vi "Element by Hierarchy.vi"(8 "error in (no error)":errorcluster, 10 "Hierarchy":string[](array[string]), 11 "Config Manager in":refnum<class "Config Manager.lvclass">) -> (0 "error out":errorcluster, 2 "Config Element":refnum<class "Config Element.lvclass">, 3 "Config Manager out":refnum<class "Config Manager.lvclass">)   [LabVIEW 2020, in "CDM-Config.lvlib" / "Config Manager.lvclass"]
doc: "Returns the specified element or an error if the specified hierarchy name does not exist. If the specified hierarchy is empty, the root element is returned."
uses:
  Config Manager.lvclass
  CDM-Config.lvlib
  Config Element/Config Element.lvclass
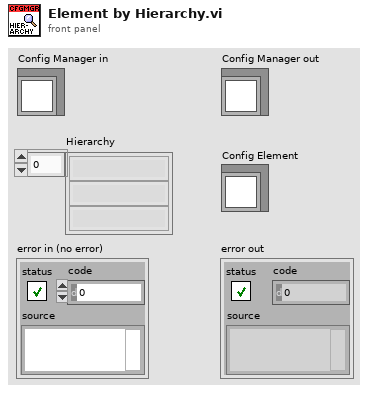
[diagram p1: front panel]
types:
  T1 = typedef "CDM-Config.lvlib/Config Manager.lvclass/Ref Data.ctl" = cluster{"Elements":refnum<class "Config Element.lvclass">[], "Hierarchy Map":map{string[], i32}, "Element Map":map{refnum<class "Config Element.lvclass">, i32}}
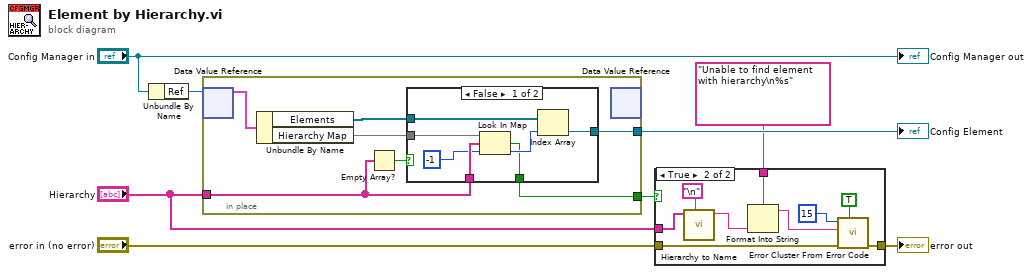
[diagram p0: block diagram]
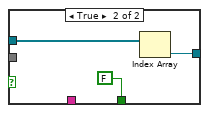
[diagram p2: hidden frame]
diagram:
  n1 = Unbundle By Name("Config Manager in") -> ("Ref"=w7:refnum<data-value>)
  n2 = in-place {
    in-place-border: "Hierarchy" -> [w9]
    in-place-border: [w12] -> w6
    in-place-border: [w11] -> w4
    n3 = in-place-dvr #1(w7) -> (w15:T1)  [unwired: 1 out]
    n4 = Unbundle By Name(w15) -> ("Elements"=w13:refnum<class "Config Element.lvclass">[], "Hierarchy Map"=w14:map{string[], i32})
    n5 = Empty Array?(array=w9) -> (empty?=w10:bool)
    n6 = case shown="False" w10 {
      tunnel: w14 -> [w22 _]
      tunnel: w13 -> [w21 w24]
      tunnel: [w19 w23] -> w12
      tunnel: [w18 FALSE ("key not found?")] -> w11
      tunnel: w9 -> [w17 _]
      frame False {
        n7 = Look In Map(map=w22, key=w17, default value=-1) -> (key not found?=w18:bool, value=w20:i32)
        n8 = Index Array(array=w21, index=w20) -> (element=w19:refnum<class "Config Element.lvclass">)
      }
      frame True {
        n9 = Index Array(array=w24) -> (element=w23:refnum<class "Config Element.lvclass">)  [unwired: 1 in]
      }
    }
    n10 = in-place-dvr #1() -> ()  [unwired: 1 in, 2 out]
  }
  "Config Element" <- w6
  n11 = case shown="True" w4 {
    tunnel: "error in (no error)" -> [w26 w34]
    tunnel: [w26 w33] -> w3
    tunnel: "Hierarchy" -> [_ w29]
    tunnel: "Unable to find element with hierarchy\n%s" -> [_ w35]
    frame False {
    }
    frame True {
      n12 = call "Hierarchy to Name.vi"("Delimiter"="\n", "Hierarchy"=w29) -> ("Full Name"=w28:string)  [unwired: 9 in]
      n13 = Format Into String(format string=w35, w28) -> (resulting string=w30:string)  [unwired: 2 in, 1 out]
      n14 = call <vilib>:"Error Cluster From Error Code.vi"("show call chain? (False)"=TRUE, "error in (no error)"=w34, "error message (\"\")"=w30, "error code (0)"=15) -> ("error out"=w33:errorcluster)  [unwired: 5 in]
    }
  }
  "error out" <- w3
  "Config Manager out" <- "Config Manager in"
